vi "Clear-reference.vi"(8 "error in (no error)":errorcluster, 10 "Data ref":T1) -> (0 "error out":errorcluster)   [LabVIEW 2013, in "PowderDeposition.lvlib" / "PD-Main.lvclass"]
uses:
  PD-Main.lvclass
  Object-reference.ctl
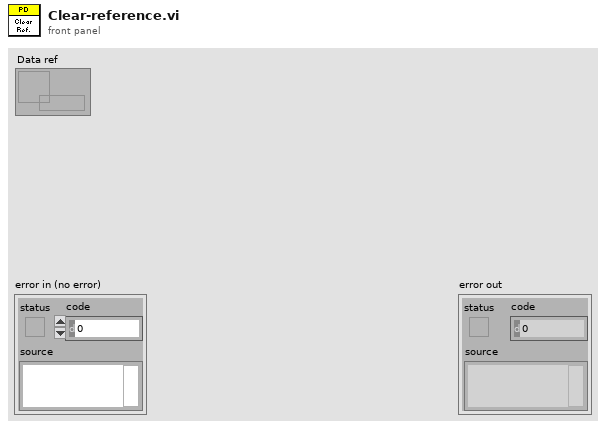
[diagram p1: front panel]
types:
  T1 = typedef "PowderDeposition.lvlib/PD-Main.lvclass/Object-reference.ctl" = refnum<data-value>
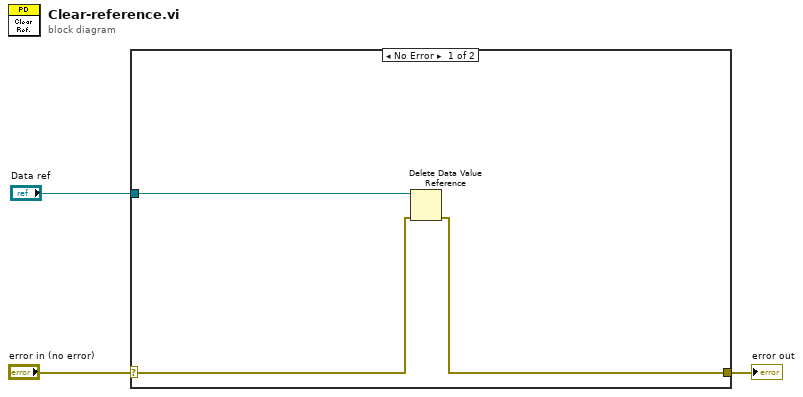
[diagram p0: block diagram]
diagram:
  n1 = case shown="No Error" "error in (no error)" {
    selector: "error in (no error)" -> [w6 w7]
    tunnel: [w5 w7] -> w2
    tunnel: "Data ref" -> [w4 _]
    frame No Error {
      n2 = Delete Data Value Reference(data value reference=w4, error in=w6) -> (error out=w5:errorcluster)  [unwired: 1 out]
    }
    frame Error {
    }
  }
  "error out" <- w2
